vi "Actor Core.vi"(8 "error in":errorcluster, 11 "Nested in":refnum<class "Test UI.lvclass">) -> (0 "error out":errorcluster, 3 "Actor out":refnum<class "Actor.lvclass">)   [LabVIEW 2024, in "Test UI.lvlib" / "Test UI.lvclass"]
doc: "(<B>Filename</B>: Actor Framework.lvlib:Actor.lvclass:Actor Core.vi)\n\nReceives messages to the actor, reacts to them, and initiates any error handling that may shut the actor down.\n\nDescendant classes may override this VI to append parallel tasks for the actor to complete while it handles messages. Overrides use the Call Parent Method node."
uses:
  Test UI.lvclass
  C:/Program Files/National Instruments/LabVIEW 2024/vi.lib/ActorFramework/Actor/Actor.lvclass
  <vilib>/ActorFramework/Actor/Actor.lvclass
  Test States/Init/Init.lvclass
  <vilib>/ActorFramework/Actor/Actor.lvclass/Actor.ctl
  <vilib>/ActorFramework/Message Enqueuer/Message Enqueuer.lvclass/Message Enqueuer.ctl
  Test UI.lvclass/Test UI.ctl
  <vilib>/ActorFramework/Message Enqueuer/Init from Existing Queue.vi
  <vilib>/ActorFramework/Message Enqueuer/Enqueue.vi
  <vilib>/ActorFramework/Stop Msg/Stop Msg.lvclass
  C:/Program Files/National Instruments/LabVIEW 2024/vi.lib/ActorFramework/Message/Message.lvclass
  Test UI Messages/Change to Idle State Msg/Change to Idle State Msg.lvclass
  <vilib>/ActorFramework/Message Priority Queue/Priority Enqueue.vi
  <vilib>/ActorFramework/Message Enqueuer/Message Enqueuer.lvclass
  Test UI Messages/Change to Work State Msg/Change to Work State Msg.lvclass
  e4eca110-b22b-4567-9fec-6f4464f3c018.vi
panel:
  in  "Start Button":bool
  out "Log":string[](array[string])
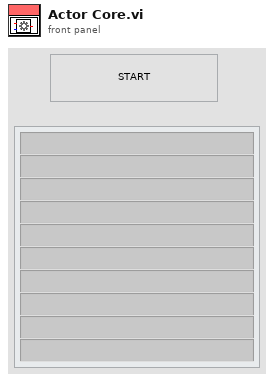
[diagram p1: front panel]
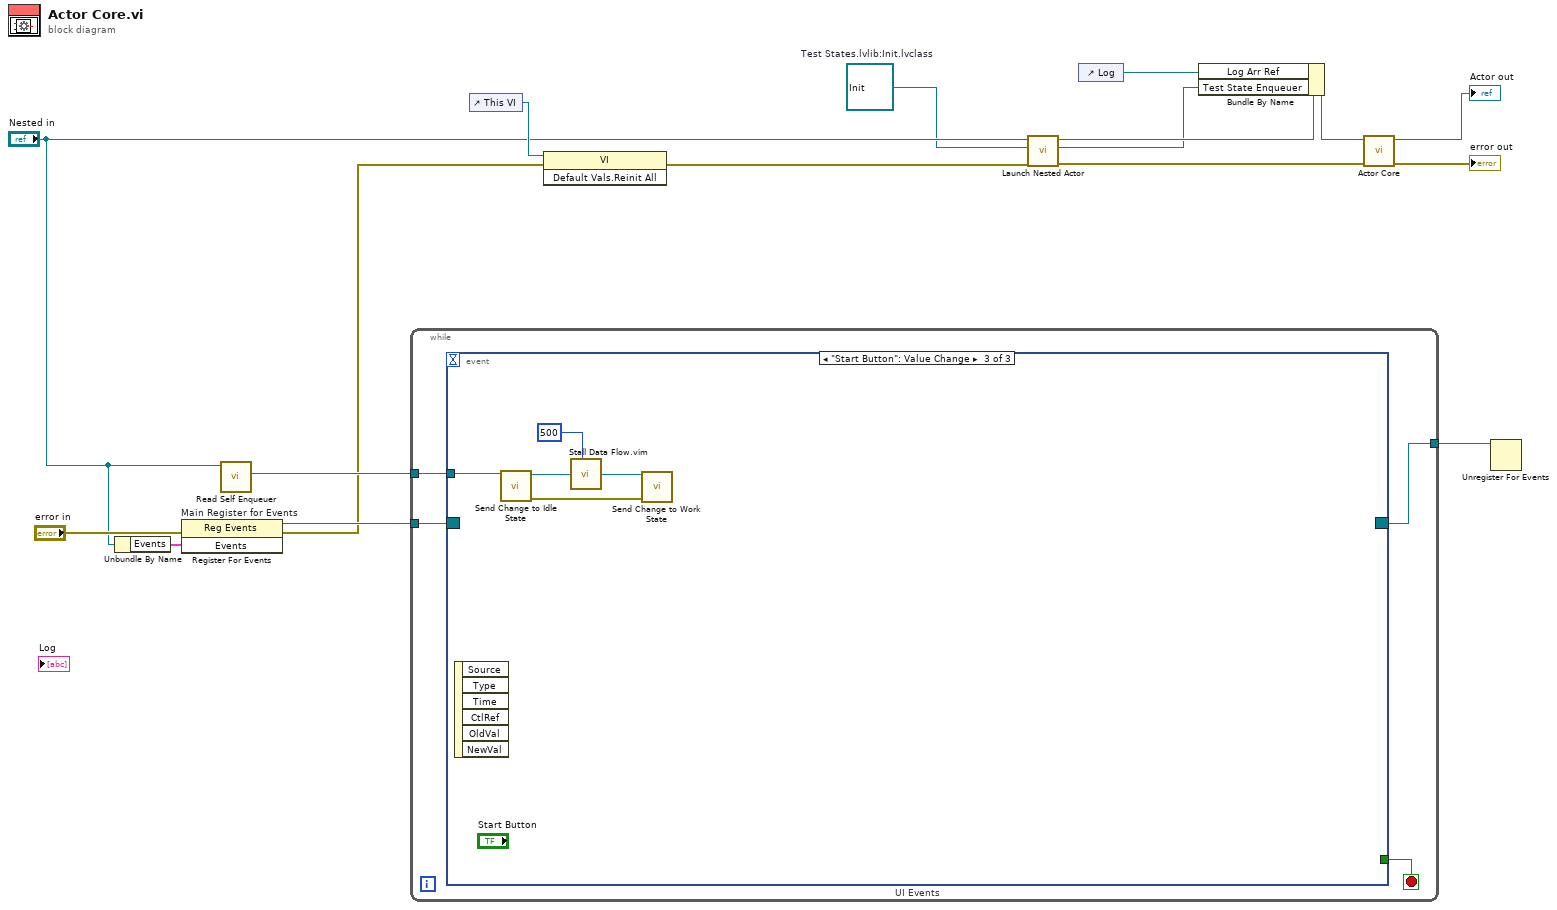
[diagram p0: block diagram]
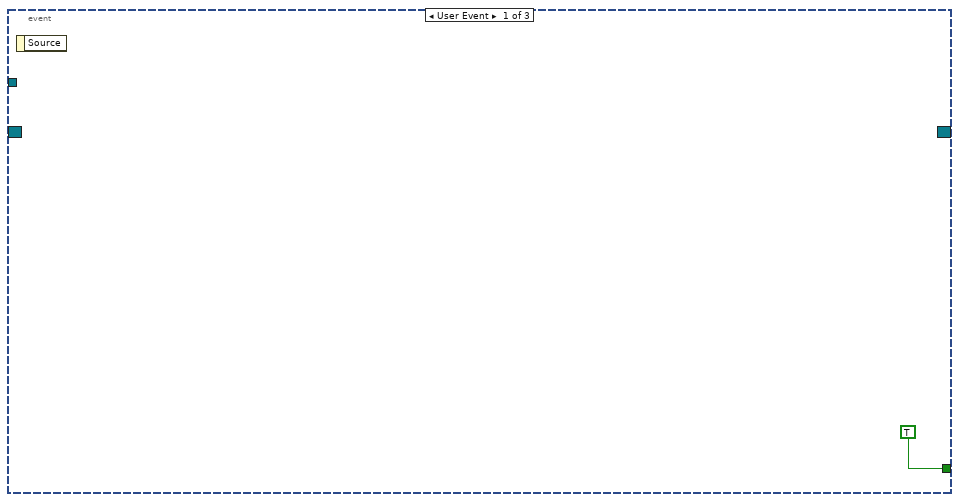
[diagram p2: hidden frame]
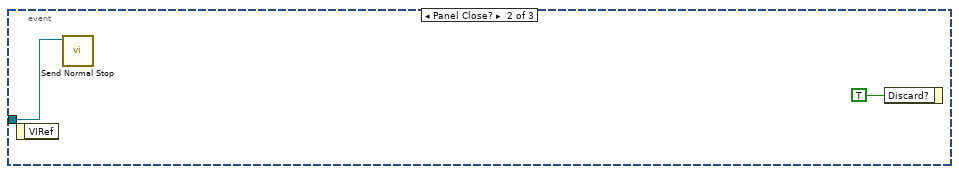
[diagram p3: hidden frame]
diagram:
  w2 = refnum<class "Init.lvclass"> refnum  # Test States.lvlib:Init.lvclass
  n1 = Unbundle By Name("Nested in") -> ("Events"=w14:cluster{"Stop":refnum<user-event>})
  n2 = register-events "Main Register for Events"(error in="error in", w14) -> (reference out=w15:refnum<event-registration>, error out=w10:errorcluster)  [unwired: 1 in]
  n3 = call <vilib>:"Read Self Enqueuer.vi"("Actor"="Nested in") -> ("Self Enqueuer"=w12:refnum<class "Message Enqueuer.lvclass">)  [unwired: 10 in]
  n4 = while {
    tunnel: w15 -> [w21]
    tunnel: [w19] -> w13
    tunnel: w12 -> [w18]
    stop <- w20 stop-if-true
    n5 = event "UI Events" shown="[2] \"Start Button\": Value Change" {
      selector: w21 -> [_ _ _]
      dyn-events: [_ _ _] -> w19
      timeout: _ -> [_ _ _]
      tunnel: [TRUE _ _] -> w20
      tunnel: w18 -> [_ w23 w29]
      event User Event {
        n6 = event-data() -> ()  [unwired: 1 in, 1 out]
      }
      event Panel Close? {
        n7 = event-data() -> ()  [unwired: 1 in, 1 out]
        n8 = call <vilib>:"Send Normal Stop.vi"("Message Enqueuer"=w23) -> ()  [unwired: 10 in, 1 out]
        n9 = event-data("Discard?"=TRUE) -> ()  [unwired: 1 in, 1 out]
      }
      event "Start Button": Value Change {
        n10 = event-data() -> ()  [unwired: 1 in, 6 out]
        n11 = call "Send Change to Idle State.vi"("Message Enqueuer"=w29) -> ("error out"=w28:errorcluster, "Message Enqueuer out"=w27:refnum<class "Message Enqueuer.lvclass">)  [unwired: 9 in]
        n12 = call "Stall Data Flow.vim"("value in"=w27, "milliseconds to wait"=u32 500) -> ("value out"=w26:refnum<class "Message Enqueuer.lvclass">)  [unwired: 1 out]
        n13 = call "Send Change to Work State.vi"("error in (no error)"=w28, "Message Enqueuer"=w26) -> ()  [unwired: 8 in, 2 out]
      }
    }
  }
  n14 = control-ref of="This VI"() -> (w8:refnum<vi>)
  n15 = invoke class="VI" method="Default Vals.Reinit All"(reference=w8, error in=w10) -> (error out=w9:errorcluster)  [unwired: 1 in, 2 out]
  n16 = call <vilib>:"Launch Nested Actor.vi"("error in (no error)"=w9, "Nested Actor"=w2, "Caller Actor in"="Nested in") -> ("error out"=w7:errorcluster, "Nested Actor's Enqueuer"=w1:refnum<class "Message Enqueuer.lvclass">, "Caller Actor out"=w6:refnum<class "Test UI.lvclass">)  [unwired: 6 in]
  n17 = control-ref of="Log"() -> (w3:refnum<vi>)
  n18 = Bundle By Name(cluster=w6, "Log Arr Ref"=w3, "Test State Enqueuer"=w1) -> (w4:refnum<class "Test UI.lvclass">)
  n19 = call-parent "Actor Core.vi"("error in"=w7, "Actor in"=w4) -> ("error out"=→"error out":errorcluster, "Actor out"=→"Actor out":refnum<class "Actor.lvclass">)  [unwired: 8 in]
  n20 = Unregister For Events(event registration refnum=w13) -> ()  [unwired: 1 in, 1 out]
